vi "ManualThresholdLocalization-2.vi"(6 "[IN] Autothreshold Images \nInstead Of Generated U8":bool, 7 "[IN] Median Filter":bool, 8 "error IN":errorcluster, 10 "[IN] Binarized Image":T2, 11 "[IN] Source Image":T2) -> (0 "error OUT":errorcluster, 2 "[OUT] X,Y Coordinates":dbl[](array[numeric]))   [LabVIEW 2020]
uses:
  <vilib>/vision/Image Controls.llb/IMAQ Image.ctl
  <vilib>/vision/NI_Vision_Development_Module.lvlib
panel:
  in  "[IN] Settings":T1={"Objects"=0, "Threshold"=128, "Reject Border"=FALSE, "Fill Holes"=FALSE, "Min Object Size"=FALSE, "Min Size"=3, "Max Object Size"=FALSE, "Max Size"=100, "Show Search Area"=FALSE, "Show Center"=TRUE, "Show Bounding Box"=TRUE} {"Objects" items=["Bright Objects", "Dark Objects"]; "Threshold" min=1 max=999999999 step=1; "Max Size" min=1 max=999999999 step=1; "Min Size" min=1 max=999999999 step=1}
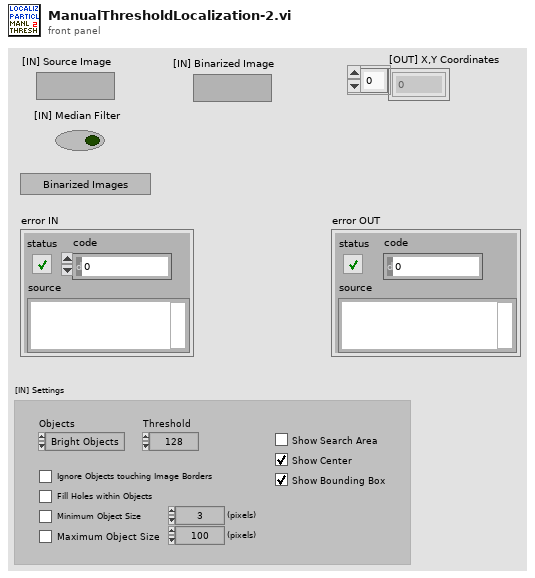
[diagram p1: front panel]
types:
  T1 = cluster{"Objects":u16, "Threshold":i32, "Reject Border":bool, "Fill Holes":bool, "Min Object Size":bool, "Min Size":i32, "Max Object Size":bool, "Max Size":i32, "Show Search Area":bool, "Show Center":bool, "Show Bounding Box":bool}
  T2 = typedef "IMAQ Image.ctl" = refnum<image>
  T3 = typedef "Image Type" = u32
  T4 = cluster{"X Size":i32, "Y Size":i32, "Order #":i32}
  T5 = cluster{"Object Center":cluster{"X":sgl, "Y":sgl}, "Bounding Box":cluster{"X Left":i32, "Y Top":i32, "X Right":i32, "Y Bottom":i32}, "Area":sgl, "Orientation":sgl, "Aspect Ratio":sgl, "Nb Holes":i32}[]
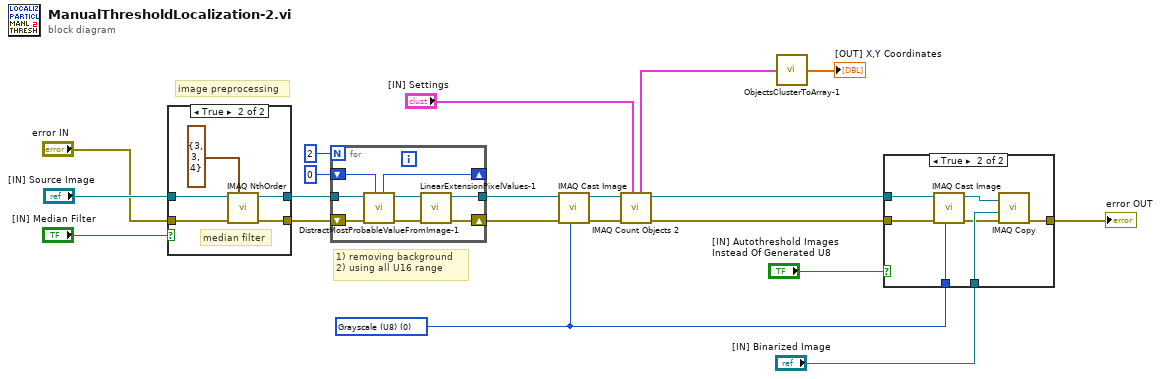
[diagram p0: block diagram]
diagram:
  w3 = T3 0 items=["Grayscale (U8)", "Grayscale (I16)", "Grayscale (SGL)", "Complex (CSG)", "RGB (U32)", "HSL (U32)", "RGB (U64)", "Grayscale (U16)"] ("Image Type")
  # "1) removing background\n2) using all U16 range"
  # "image preprocessing"
  n1 = case shown="True" "[IN] Median Filter" {
    tunnel: "[IN] Source Image" -> [w22 w26]
    tunnel: "error IN" -> [w21 w25]
    tunnel: [w22 w24] -> w8
    tunnel: [w21 w23] -> w7
    frame False {
    }
    frame True {
      # "median filter"
      n2 = call "IMAQ NthOrder"("Image Src"=w26, "Size & Order #"=T4 {"X Size"=3, "Y Size"=3, "Order #"=4}, "error in (no error)"=w25) -> ("Image Dst Out"=w24:T2, "error out"=w23:errorcluster)  [unwired: 4 in]
    }
  }
  n3 = for {
    N: 2 -> [_]
    shift-right: [w29] -> w4
    shift-left: w7 -> [w33]
    shift-right: [w28] -> _
    shift-left: 0 ("[IN] # Iteration") -> [w35]
    tunnel: w8 -> [w34]
    tunnel: [w30] -> w5
    n4 = call "DistractMostProbableValueFromImage-1.vi"("[IN] # Iteration"=w35, "error in"=w33, "[IN] Max Projected Image"=w34) -> ("error out"=w31:errorcluster, "[OUT] Processed Image"=w32:T2, "[OUT] # Iteration"=w28:i32)  [unwired: 6 in]
    n5 = call "LinearExtensionPixelValues-1.vi"("error in"=w31, "[IN] Max Projected Image"=w32) -> ("error out"=w29:errorcluster, "[OUT] Processed Image"=w30:T2)  [unwired: 8 in]
  }
  n6 = call "IMAQ Cast Image"("Image Type"=w3, "error in (no error)"=w4, "Image Src"=w5) -> ("error out"=w1:errorcluster, "Image Dst Out"=w2:T2)  [unwired: 7 in]
  n7 = call "IMAQ Count Objects 2"("Settings"="[IN] Settings", "error in (no error)"=w1, "Image"=w2) -> ("error out"=w15:errorcluster, "Image Out"=w14:T2, "Objects"=w11:T5)  [unwired: 4 in, 2 out]
  n8 = call "ObjectsClusterToArray-1.vi"("[IN] Objects"=w11) -> ("[OUT] X,Y Coordinates"=→"[OUT] X,Y Coordinates":dbl[])
  n9 = case shown="True" "[IN] Autothreshold Images \nInstead Of Generated U8" {
    tunnel: w15 -> [w36 w42]
    tunnel: [w36 w43] -> w12
    tunnel: w14 -> [_ w41]
    tunnel: w3 -> [_ w40]
    tunnel: "[IN] Binarized Image" -> [_ w38]
    frame False {
    }
    frame True {
      n10 = call "IMAQ Cast Image"("Image Type"=w40, "error in (no error)"=w42, "Image Src"=w41) -> ("error out"=w37:errorcluster, "Image Dst Out"=w39:T2)  [unwired: 7 in]
      n11 = call "IMAQ Copy"("error in (no error)"=w37, "Image Dst"=w38, "Image Src"=w39) -> ("error out"=w43:errorcluster)  [unwired: 3 in, 1 out]
    }
  }
  "error OUT" <- w12
